vi "PanelDiagramShortcuts.vi"() -> ()   [LabVIEW 2019]
doc: "This updates the <b><labview>\\LabVIEW.ini</b> using Ryan's Quick Drop Block Diagram and Panel shortcuts.\n\nCreated by: Ryan Pacini"
panel:
  in  "Panel Shortcuts":string="ac:Array;\nb:Push Button;\nbb:Round LED;\nc:Cluster;\nd:Numeric Control;\ndd:Numeric Indicator;\ne:Enum;\ner:Error In 3D.ctl;\nerr:Error Out 3D.ctl;\np:File Path Control;\npp:File Path Indicator;\ns:String Control;\nss:String Indicator;\nt:Time Stamp Control;\ntt:Time Stamp Indicator;\nv:Variant;\nvi:VI Refnum;\nvisa:VISA resource name;"
  in  "Diagram Shortcuts":string="!=0:Not Equal To 0?;\n!=:Not Equal?;\n':Empty String/Path?;\n<0:Less Than 0?;\n<:Less?;\n<=0:Less Or Equal To 0?;\n<=:Less Or Equal?;\n=0:Equal To 0?;\n=:Equal?;\n>0:Greater Than 0?;\n>:Greater?;\n>=0:Greater Or Equal To 0?;\n>=:Greater Or Equal?;\na:Build Array;\naa:Index Array;\nac:Array Constant;\nad:Delete From Array;\nar:Replace Array Subset;\nb:Bundle By Name;\nbb:False Constant;\nbu:Build Path;\nc:Cluster Constant;\ncase:Case Structure;\ncdb:To Double Precision Complex;\ncl:Close Reference;\ncsg:To Single Precision Complex;\ncxt:To Extended Precision Complex;\nd:Numeric Constant;\ndbl:To Double Precision Float;\ndia:Diagram Disable Structure;\ne:Enum Constant;\next:To Extended Precision Float;\nf:Format Into String;\nfor:For Loop;\nfs:Flatten To String;\ni16:To Word Integer;\ni32:To Long Integer;\ni64:To Quad Integer;\ni8:To Byte Integer;\ni:Invoke Node;\nin:In Place Element Structure;\nmer:Merge Errors;\nms:Wait (ms);\nnan:Not A Number/Path/Refnum?;\nop:Open VI Reference;\np:Property Node;\npp:Path Constant;\ns:String Constant;\nsc:Scan From String;\nse:Select;\nsgl:To Single Precision Float;\nt:Time Stamp Constant;\nthis:VI Server Reference;\nu16:To Unsigned Word Integer;\nu32:To Unsigned Long Integer;\nu64:To Unsigned Quad Integer;\nu8:To Unsigned Byte Integer;\nu:Unbundle By Name;\nun:Unflatten From String;\nv:Variant To Data;\nvc:Variant Constant;\nwh:While Loop;"
  # "Instructions:\n1. Run this VI to replace Ryan's Quick Drop Panel & Diagram Shortcuts\n     in the '<LabVIEW>\\LabVIEW.ini' configuration file\n2. Restart LabVIEW"
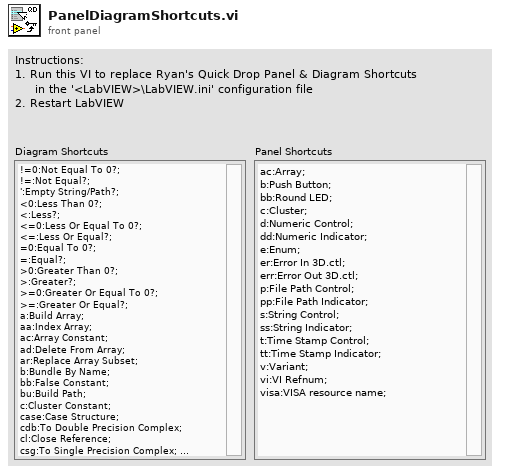
[diagram p1: front panel]
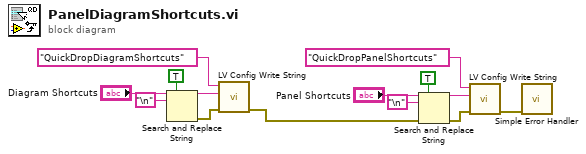
[diagram p0: block diagram]
diagram:
  n1 = Search and Replace String(replace all?=TRUE ("replace all? (F)"), input string="Diagram Shortcuts", search string="\n") -> (result string=w9:string, error out=w8:errorcluster)  [unwired: 5 in, 2 out]
  n2 = call <resource>:"LV Config Write String.vi"("error in (no error)"=w8, "value"=w9, "key"="QuickDropDiagramShortcuts") -> ("error out"=w5:errorcluster)  [unwired: 4 in]
  n3 = Search and Replace String(replace all?=TRUE ("replace all? (F)"), input string="Panel Shortcuts", search string="\n", error in=w5) -> (result string=w3:string, error out=w4:errorcluster)  [unwired: 4 in, 2 out]
  n4 = call <resource>:"LV Config Write String.vi"("error in (no error)"=w4, "value"=w3, "key"="QuickDropPanelShortcuts") -> ("error out"=w1:errorcluster)  [unwired: 4 in]
  n5 = call <vilib>:"Simple Error Handler.vi"("error in (no error)"=w1) -> ()  [unwired: 4 in, 5 out]
